vi "DI Block Config Pane.vi"(6 "_SubPanelMessages":refnum<notifier>, 9 "_myEmbeddedToFrameEvent":T7, 10 "_myEmbedded.Exit":refnum<user-event>, 11 "-Property Bundle":cluster{"Name":string, "Value":variant}[](array[cluster])) -> (1 "_Connection Informations":T3, 2 "_Scripter Input":T9)   [LabVIEW 2021]
doc: "Reads values from one or more digital input channels. Use this Express VI to read one or multiple samples for each channel at one time."
uses:
  <vilib>/myRIO/Common/Express VI Framework/xctls/myRIO Channel List/myRIO Channel List.xctl
  <vilib>/myRIO/Common/Express VI Framework/typedefs/Config Pane to Framework Ref.ctl
  <vilib>/myRIO/Common/Express VI Framework/typedefs/Data Validate Ref.ctl
  <vilib>/myRIO/Common/Express VI Framework/typedefs/Scripter Input.ctl
  <vilib>/myRIO/Common/Express VI Framework/typedefs/WireThrough Terminal Names.ctl
  <vilib>/myRIO/Common/Express VI Framework/typedefs/Instrument Driver Method Descriptor Array.ctl
  <vilib>/myRIO/Common/Express VI Framework/typedefs/Instrument Driver Method Descriptor.ctl
  <vilib>/myRIO/Common/Express VI Framework/typedefs/Sub Panel Messages.ctl
  <vilib>/myRIO/Common/Express VI Framework/typedefs/Connection Informations.ctl
  <vilib>/myRIO/Common/Instrument Driver Framework/Utilities/typedefs/Channel Types.ctl
  <vilib>/myRIO/Common/Express VI Framework/vis/Express VI Framework Strings Global.vi
panel:
  out "_learnMoreLatency":string="Gaps exist between sequential n samples acquisitions Learn more"
  out "_learnMoreFrequency":string="Detailed information about valid sample rates for this Express VI.  Learn more"
  in  "_Validate":bool
  in  "Sample Rate:":dbl=1.0 caption="Sample rate:"
  in  "Sample Rate Unit":enum16{"kHz", "MHz"}(ring)
  in  "Samples to Read:":u32=1000 caption="Samples:" min=1 max=10000
  in  "Name:":string="Digital input (n samples)" caption="Node name:"
  in  "Selected Channel List":T1[](xcontrol)=[{"Channel Name"=0, "Channel Alias"="", "Remove Channel"=FALSE, "Index"=0}]
  in  "_Default Alias String":string
  in  "_VI Default Name (Edit and make value default)":string="Digital input (n samples)"
  in  "_WireThrough Info (Edit and make value default)":T4={"WireThrough Top In"="DI (N Samples) Ref In", "WireThrough Bottom In"="error in (no error)", "WireThrough Top Out"="DI (N Samples) Ref Out", "WireThrough Bottom Out"="error out"}
  in  "_Template Array (Edit and make value default)":T5=[{"Function Name"="Smart Open", "VI Path"=path "<vilib>/myRIO/Instrument Drivers/Onboard IO/DI Block/vis", "Script"=TRUE, "Inputs"=[{"name"="Channel Names", "value"=variant, "Config Pane Only"=TRUE, "Build Array"=FALSE, "Bundle Cluster"=FALSE, "Show Term"=FALSE, "alias"=[], "Required Input"=FALSE}], "Outputs"=[], "VI Class"=enum."Open", "Controls Refs[]"=[], "Inline"=FALSE}, {"Function Name"="Open", "VI Path"=path "<vilib>/myRIO/Instrument Drivers/Onboard IO/DI Block/vis", "Script"=FALSE, "Inputs"=[{"name"="Channel Names", "value"=variant, "Config Pane Only"=TRUE, "Build Array"=FALSE, "Bundle Cluster"=FALSE, "Show Term"=FALSE, "alias"=[], "Required Input"=FALSE}], "Outputs"=[], "VI Class"=enum."Open", "Controls Refs[]"=[], "Inline"=FALSE}, {"Function Name"="Read", "VI Path"=path "<vilib>/myRIO/Instrument Drivers/Onboard IO/DI Block/vis", "Script"=TRUE, "Inputs"=[{"name"="Number of Samples", "value"=variant, "Config Pane Only"=TRUE, "Build Array"=FALSE, "Bundle Cluster"=FALSE, "Show Term"=FALSE, "alias"=[], "Required Input"=FALSE}, {"name"="Sample Rate [Hz]", "value"=variant, "Config Pane Only"=TRUE, "Build Array"=FALSE, "Bundle Cluster"=FALSE, "Show Term"=FALSE, "alias"=[], "Required Input"=FALSE}], "Outputs"=[{"name"="Values", "value"=variant, "Show Term"=TRUE, "Index Array"=TRUE, "Unbundle Cluster"=FALSE, "alias"=[]}], "VI Class"=enum."Data", "Controls Refs[]"=[], "Inline"=FALSE}, {"Function Name"="Close", "VI Path"=path "<vilib>/myRIO/Instrument Drivers/Onboard IO/DI Block/vis", "Script"=FALSE, "Inputs"=[], "Outputs"=[], "VI Class"=enum."Close", "Controls Refs[]"=[], "Inline"=FALSE}]
  in  "_Test Close":bool
  # "User Visible Area"
  # "NOTE: Tab Order has been set\nfor this Front Panel.\n1. Name: (string control)\n2. Add Channel (button)\n3. Selected Channel List (array)\n\nAll other controls are excluded \nfrom Tabbing order\n\nTo exlude a control from context\nhelp prefix its label text with a '-'"
  # "Gap:"
  # "Acquired signal"
  # "Missed signal"
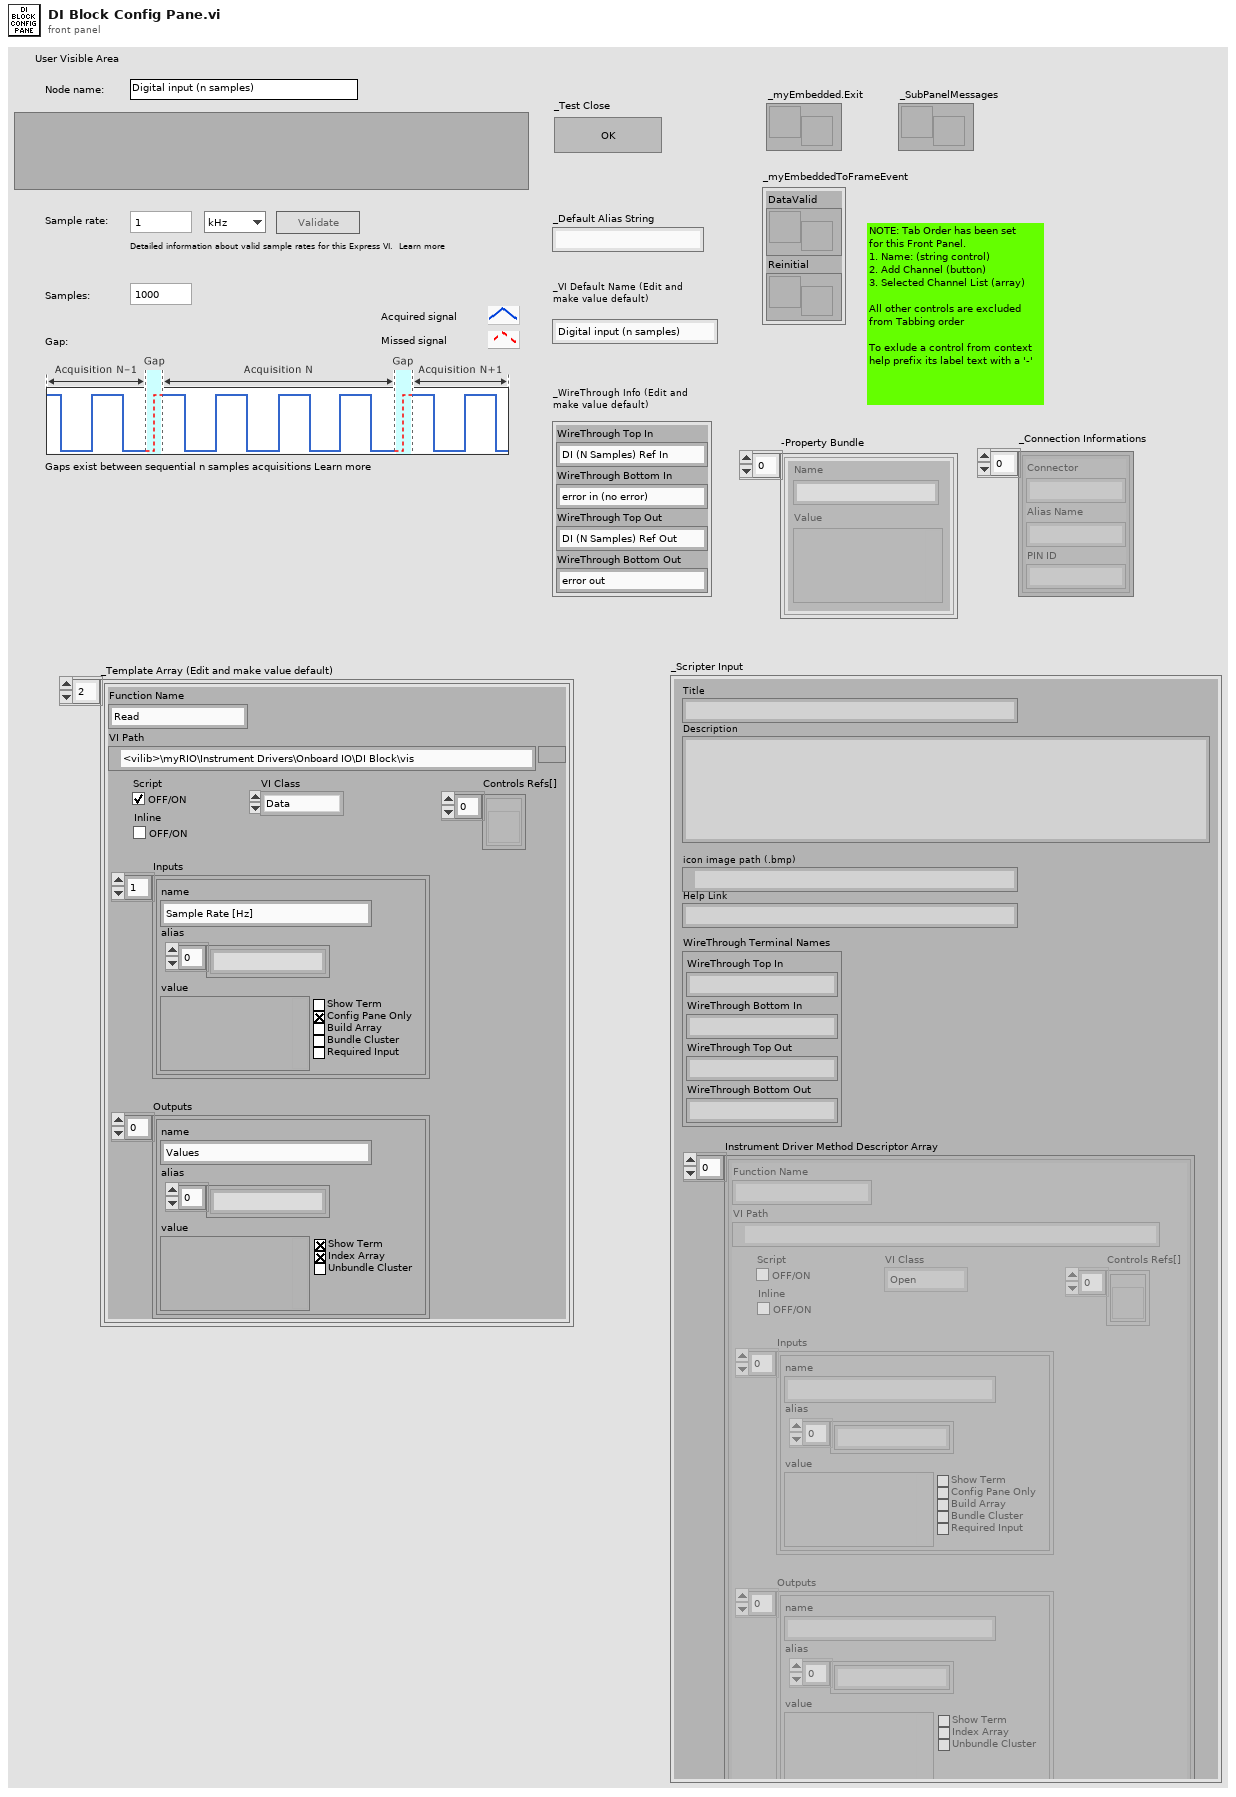
[diagram p1: front panel]
types:
  T1 = typedef "myRIO Channel List.xctl/Channel Data.ctl" = cluster{"Channel Name":u16, "Channel Alias":string, "Remove Channel":T2, "Index":i32}
  T2 = typedef "myRIO Channel List.xctl/Remove Channel.ctl" = bool
  T3 = typedef "Connection Informations.ctl" = cluster{"Connector":string, "Alias Name":string, "PIN ID":string}[]
  T4 = typedef "WireThrough Terminal Names.ctl" = cluster{"WireThrough Top In":string, "WireThrough Bottom In":string, "WireThrough Top Out":string, "WireThrough Bottom Out":string}
  T5 = typedef "Instrument Driver Method Descriptor Array.ctl" = T6[]
  T6 = typedef "Instrument Driver Method Descriptor.ctl" = cluster{"Function Name":string, "VI Path":path, "Script":bool, "Inputs":cluster{"name":string, "value":variant, "Config Pane Only":bool, "Build Array":bool, "Bundle Cluster":bool, "Show Term":bool, "alias":string[], "Required Input":bool}[], "Outputs":cluster{"name":string, "value":variant, "Show Term":bool, "Index Array":bool, "Unbundle Cluster":bool, "alias":string[]}[], "VI Class":enum16{"Open", "Configure", "Data", "Manage", "Close"}, "Controls Refs[]":refnum<vi>[], "Inline":bool}
  T7 = typedef "Config Pane to Framework Ref.ctl" = cluster{"DataValid":T8, "Reinitial":refnum<user-event>}
  T8 = typedef "Data Validate Ref.ctl" = refnum<user-event>
  T9 = typedef "Scripter Input.ctl" = cluster{"Title":string, "Description":string, "icon image path (.bmp)":path, "Help Link":string, "WireThrough Terminal Names":T4, "Instrument Driver Method Descriptor Array":T5}
  T10 = typedef "Channel Types.ctl" = enum32{"Unknown", "AI", "AO", "DIO - DI", "DIO", "DIO - DO", "I2C", "PWM", "Encoder", "SPI", "UART", "Accelerometer", "DIO - LED", "DIO - Button", "AI (N Samples)", "AudioIn (N Samples)", "AO (N Samples)", "AudioOut (N Samples)", "DI (N Samples)", "DO (N Samples)", "AI IRQ", "DI IRQ", "Timer IRQ", "RSL", "Relay", "CAN", "AI (Continuous)", "AO (Continuous)"}
  T11 = typedef "Channel Info.ctl" = cluster{"Channel Name":string, "Alias":string, "Used?":bool, "Not Support?":bool, "Property Bundle":cluster{"Name":string, "Value":variant}[]}
  T12 = typedef "Sub Panel Messages.ctl" = enum16{"Initialized"}
  T13 = enum8{"Enabled", "Disabled", "Disabled and Grayed Out"}
  T14 = cluster{"Connector":string, "Alias Name":string, "PIN ID":string}[]
  T15 = cluster{"name":string, "value":variant, "Config Pane Only":bool, "Build Array":bool, "Bundle Cluster":bool, "Show Term":bool, "alias":string[], "Required Input":bool}[]
  T16 = cluster{"name":string, "value":variant, "Config Pane Only":bool, "Build Array":bool, "Bundle Cluster":bool, "Show Term":bool, "alias":string[], "Required Input":bool}
  T17 = cluster{"name":string, "value":variant, "Show Term":bool, "Index Array":bool, "Unbundle Cluster":bool, "alias":string[]}[]
  T18 = cluster{"name":string, "value":variant, "Show Term":bool, "Index Array":bool, "Unbundle Cluster":bool, "alias":string[]}
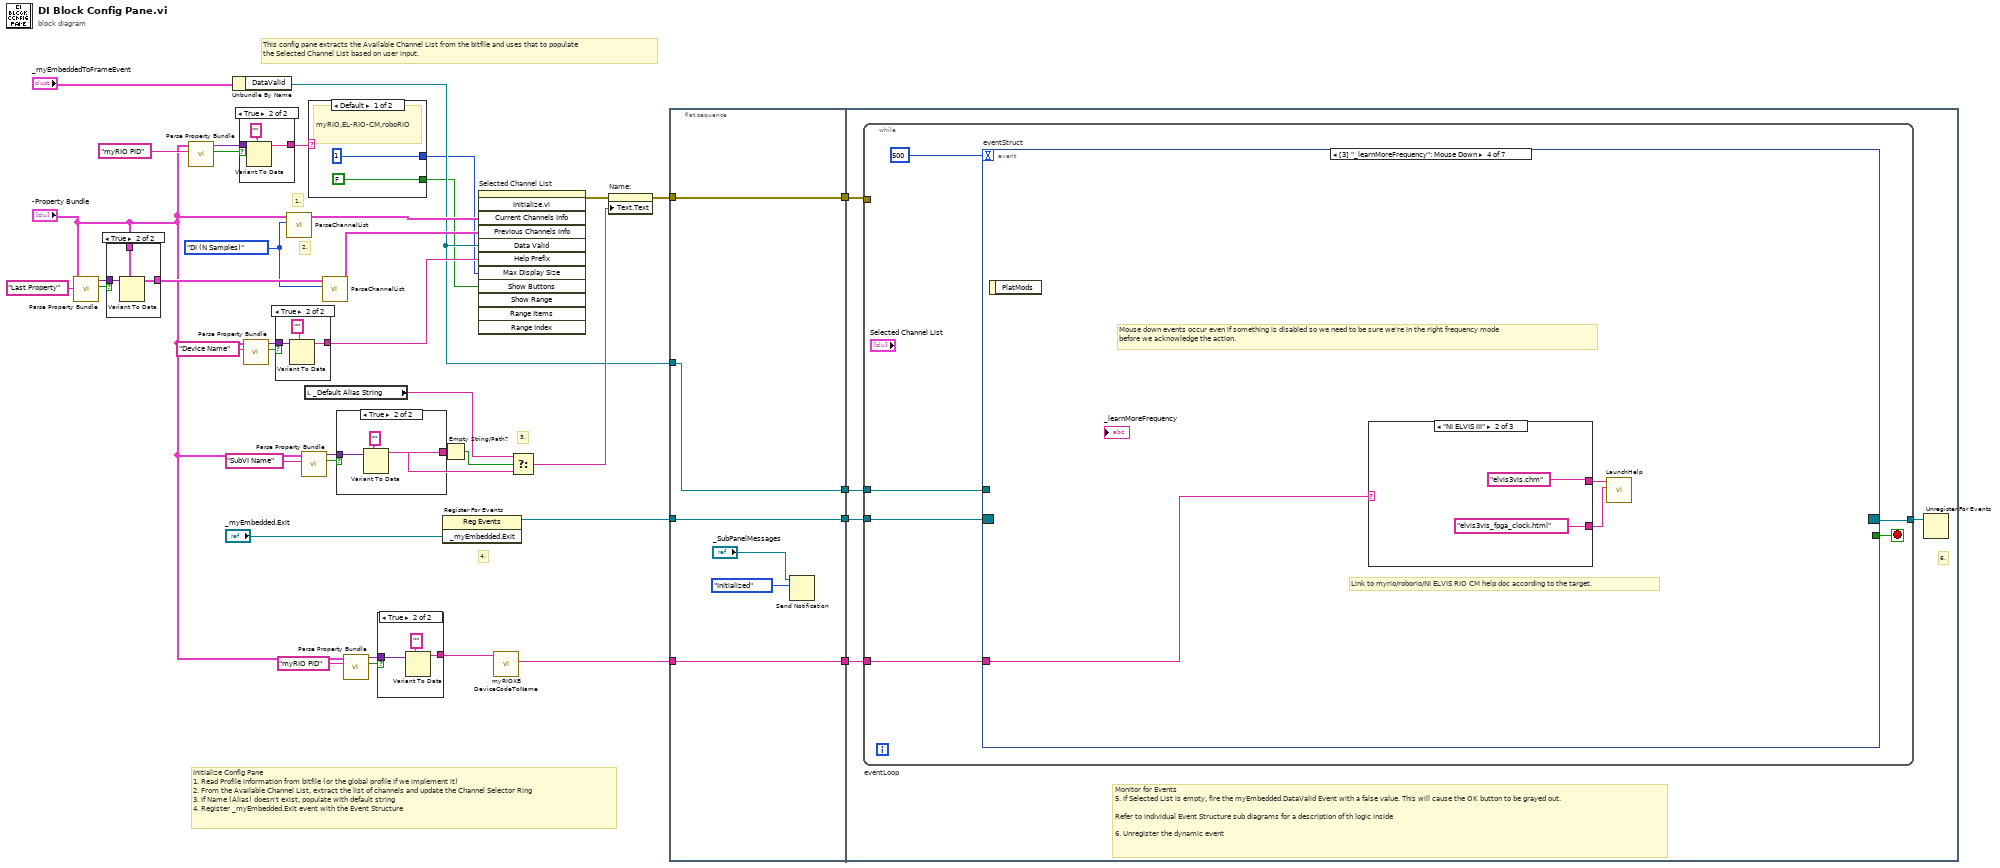
[diagram p0: block diagram]
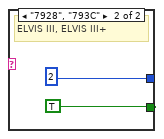
[diagram p2: hidden frame]
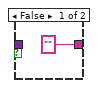
[diagram p3: hidden frame]
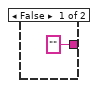
[diagram p4: hidden frame]
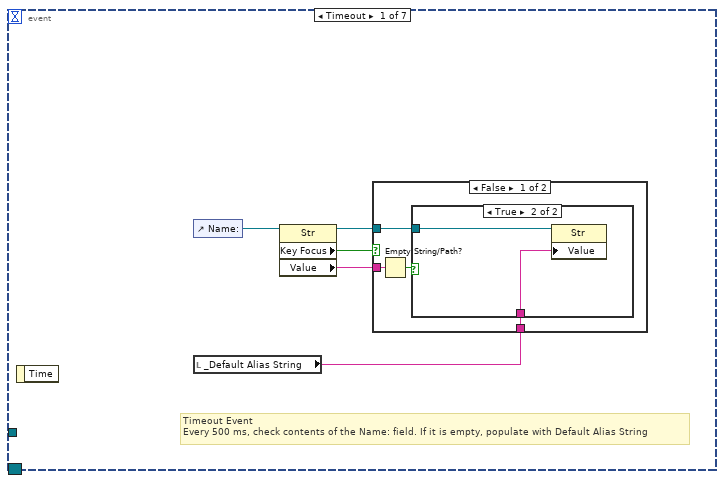
[diagram p5: hidden frame]
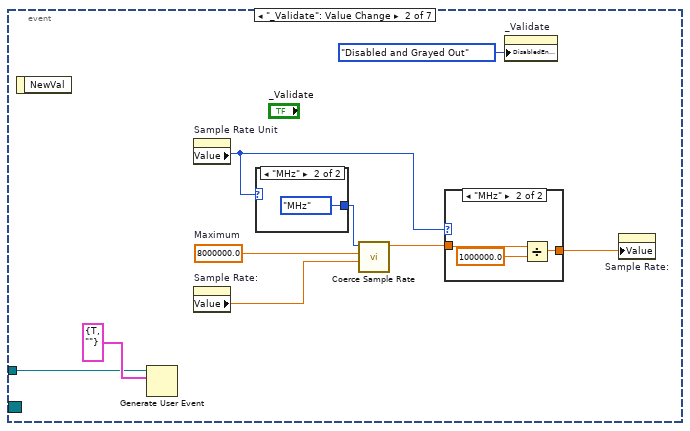
[diagram p8: hidden frame]
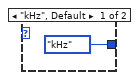
[diagram p9: hidden frame]
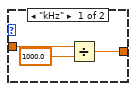
[diagram p10: hidden frame]
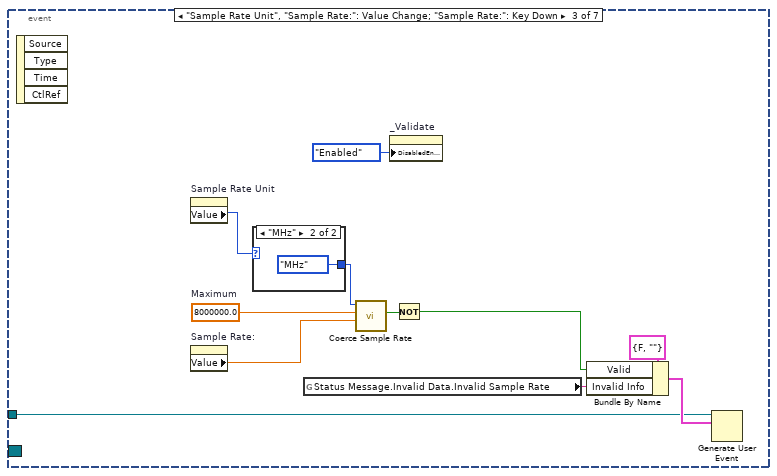
[diagram p11: hidden frame]
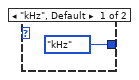
[diagram p12: hidden frame]
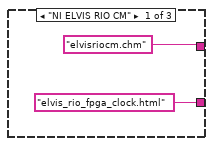
[diagram p13: hidden frame]
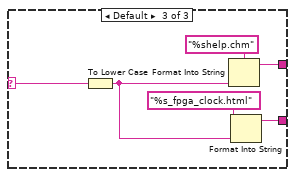
[diagram p14: hidden frame]
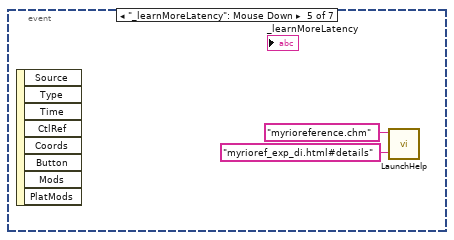
[diagram p15: hidden frame]
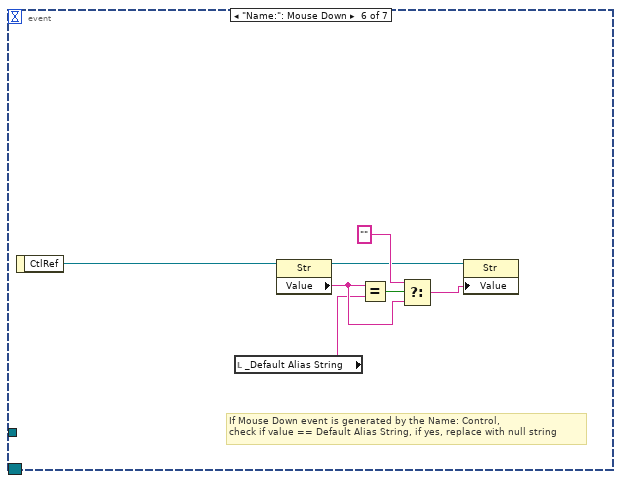
[diagram p16: hidden frame]
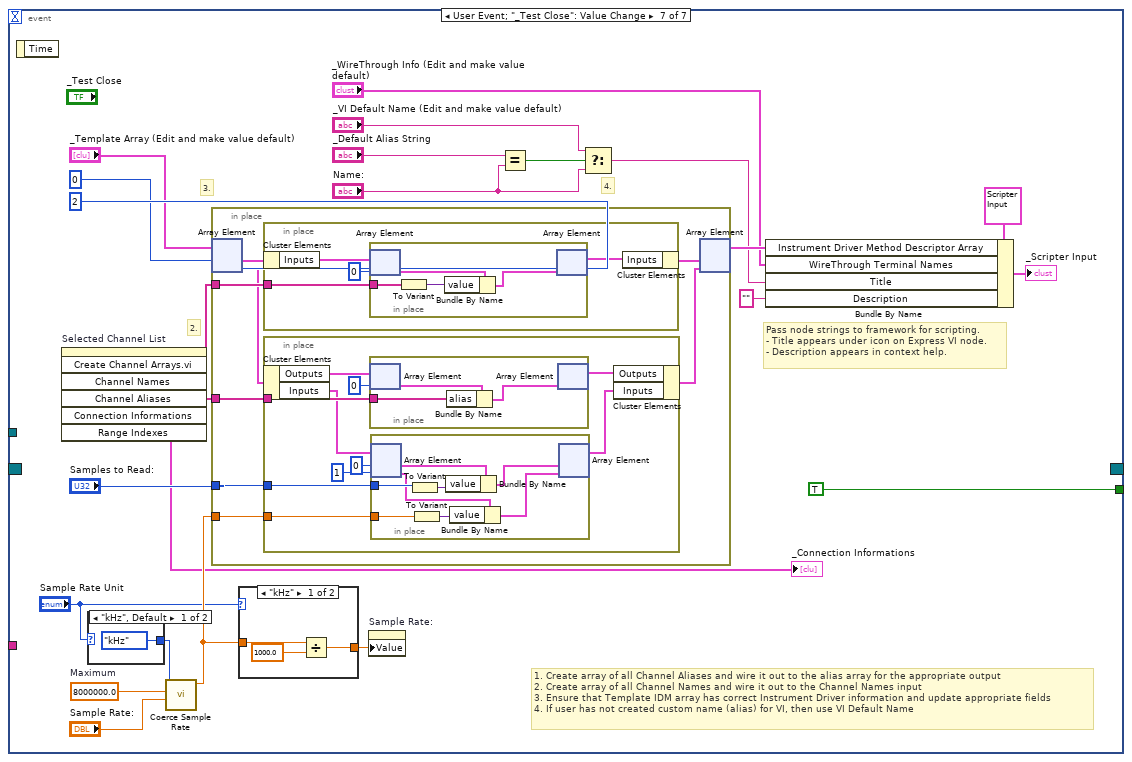
[diagram p17: hidden frame]
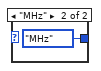
[diagram p18: hidden frame]
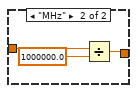
[diagram p19: hidden frame]
diagram:
  w24 = Channel_Types."DI (N Samples)" ("Channel to Read")
  # "This config pane extracts the Available Channel List from the bitfile and uses that to populate\nthe Selected Channel List based on user input."
  # "2."
  # "1."
  # "4."
  # "3."
  # "Initialize Config Pane\n1. Read Profile information from bitfile (or the global profile if we implement it)\n2. From the Available Channel List, extract the list of channels and update the Channel Selector Ring\n3. If Name (Alias) doesn't exist, populate with default string\n4. Register _myEmbedded.Exit event with the Event Structure"
  n1 = call <vilib>:"Parse Property Bundle.vi"("Name"="Last Property", "Property Bundle"="-Property Bundle") -> ("Found?"=w26:bool, "Value"=w27:variant)  [unwired: 8 in]
  n2 = case shown="True" w26 {
    tunnel: w27 -> [_ w43]
    tunnel: [_ w42] -> w25
    tunnel: "-Property Bundle" -> [_ w41]
    frame False {
    }
    frame True {
      n3 = Variant To Data(type=w41, Variant=w43) -> (data=w42:cluster{"Name":string, "Value":variant}[])  [unwired: 1 in, 1 out]
    }
  }
  n4 = call <vilib>:"Parse Property Bundle.vi"("Name"="myRIO PID", "Property Bundle"="-Property Bundle") -> ("Found?"=w5:bool, "Value"=w6:variant)  [unwired: 8 in]
  n5 = Unbundle By Name("_myEmbeddedToFrameEvent") -> ("DataValid"=w15:T8)
  n6 = case shown="True" w5 {
    tunnel: w6 -> [_ w47]
    tunnel: ["" ("Name") w46] -> w4
    frame False {
    }
    frame True {
      n7 = Variant To Data(type="" ("Name"), Variant=w47) -> (data=w46:string)  [unwired: 1 in, 1 out]
    }
  }
  n8 = call <vilib>:"Parse Property Bundle.vi"("Name"="Device Name", "Property Bundle"="-Property Bundle") -> ("Found?"=w21:bool, "Value"=w20:variant)  [unwired: 8 in]
  n9 = case shown="True" w21 {
    tunnel: w20 -> [_ w50]
    tunnel: [_ w49] -> w19
    frame False {
    }
    frame True {
      n10 = Variant To Data(type="", Variant=w50) -> (data=w49:string)  [unwired: 1 in, 1 out]
    }
  }
  n11 = call <vilib>:"ParseChannelList.vi"("Channel to Read"=w24, "_Property Bundle"="-Property Bundle") -> ("Channel List Out"=w29:T11[])  [unwired: 7 in, 2 out]
  n12 = call <vilib>:"Parse Property Bundle.vi"("Name"="SubVI Name", "Property Bundle"="-Property Bundle") -> ("Found?"=w34:bool, "Value"=w35:variant)  [unwired: 8 in]
  n13 = local read "_Default Alias String"() -> (w30:string)
  n14 = case shown="Default" w4 {
    tunnel: [FALSE TRUE] -> w2
    tunnel: [1 ("Max Display Size") 2 ("Max Display Size")] -> w1
    frame Default {
      # "myRIO,EL-RIO-CM,roboRIO"
    }
    frame "7928", "793C" {
      # "ELVIS III, ELVIS III+"
    }
  }
  n15 = call <vilib>:"ParseChannelList.vi"("Channel to Read"=w24, "_Property Bundle"=w25) -> ("Channel List Out"=w23:T11[])  [unwired: 7 in, 2 out]
  n16 = case shown="True" w34 {
    tunnel: w35 -> [_ w58]
    tunnel: ["" ("Name") w56] -> w33
    frame False {
    }
    frame True {
      n17 = Variant To Data(type="" ("Name"), Variant=w58) -> (data=w56:string)  [unwired: 1 in, 1 out]
    }
  }
  n18 = call <vilib>:"Parse Property Bundle.vi"("Name"="myRIO PID", "Property Bundle"="-Property Bundle") -> ("Found?"=w11:bool, "Value"=w12:variant)  [unwired: 8 in]
  n19 = case shown="True" w11 {
    tunnel: w12 -> [_ w62]
    tunnel: ["" ("Name") w60] -> w8
    frame False {
    }
    frame True {
      n20 = Variant To Data(type="" ("Name"), Variant=w62) -> (data=w60:string)  [unwired: 1 in, 1 out]
    }
  }
  n21 = register-events("_myEmbedded.Exit") -> (reference out=w32:refnum<event-registration>)  [unwired: 2 in, 1 out]
  n22 = Empty String/Path?(string/path=w33) -> (empty?=w39:bool)
  n23 = invoke on="Selected Channel List" class="myRIO Channel List (strict)" method="Initialize.vi"("Current Channels Info"=w29, "Previous Channels Info"=w23, "Data Valid"=w15, "Help Prefix"=w19, "Max Display Size"=w1, "Show Buttons"=w2) -> (error out=w31:errorcluster)  [unwired: 6 in, 11 out]
  n24 = call <vilib>:"myRIOXB DeviceCodeToName.vi"("Device Code"=w8) -> ("Name"=w9:string)  [unwired: 10 in]
  n25 = Select(t=w30, s=w39, f=w33) -> (s? t:f=w38:string)
  n26 = property on="Name:" class="Str"(error in=w31, "Text.Text"=w38) -> (error out=w37:errorcluster)  [unwired: 1 in, 1 out]
  n27 = flat-sequence {
    tunnel: w32 -> [w67]
    tunnel: w37 -> [w68]
    tunnel: [w68] -> w17
    tunnel: [w67] -> w16
    tunnel: w15 -> [w64]
    tunnel: [w64] -> w14
    tunnel: w9 -> [w63]
    tunnel: [w63] -> w10
    tunnel: w17 -> [w72]
    tunnel: w16 -> [w71]
    tunnel: w14 -> [w70]
    tunnel: w10 -> [w69]
    frame #0 {
      n28 = Send Notification(notification=Sub_Panel_Messages."Initialized", notifier="_SubPanelMessages") -> ()  [unwired: 1 in, 2 out]
    }
    frame #1 {
      # "6."
      # "Monitor for Events\n5. If Selected List is empty, fire the myEmbedded.DataValid Event with a false value. This will cause the OK button to be grayed out.\n\nRefer to individual Event Structure sub diagrams for a description of th logic inside\n\n6. Unregister the dynamic event"
      n29 = while "eventLoop" {
        tunnel: w71 -> [w78]
        tunnel: [w77] -> w73
        tunnel: w72 -> [_]
        tunnel: w70 -> [w75]
        tunnel: w69 -> [w74]
        stop <- w79 stop-if-true
        n30 = event "eventStruct" shown="[3] \"_learnMoreFrequency\": Mouse Down" {
          selector: w78 -> [_ _ _ _ _ _ _]
          dyn-events: [_ _ _ _ _ _ _] -> w77
          timeout: 500 -> [_ _ _ _ _ _ _]
          tunnel: [_ _ _ _ _ _ TRUE ("_Test Close")] -> w79
          tunnel: w75 -> [_ w91 w110 _ _ _ _]
          tunnel: w74 -> [_ _ _ w121 _ _ _]
          event Timeout {
            # "Timeout Event\nEvery 500 ms, check contents of the Name: field. If it is empty, populate with Default Alias String"
            n31 = event-data() -> ()  [unwired: 1 in, 1 out]
            n32 = control-ref of="Name:"() -> (w82:refnum<vi>)
            n33 = local read "_Default Alias String"() -> (w80:string)
            n34 = property on="Property Node" class="Str"(reference=w82) -> (reference out=w81:refnum<vi>, "Key Focus"=w83:bool, "Value"=w84:string)  [unwired: 1 in, 1 out]
            n35 = case shown="False" w83 {
              tunnel: w84 -> [w88 _]
              tunnel: w81 -> [w86 _]
              tunnel: w80 -> [w85 _]
              frame False {
                n36 = Empty String/Path?(string/path=w88) -> (empty?=w87:bool)
                n37 = case shown="True" w87 {
                  tunnel: w86 -> [_ w90]
                  tunnel: w85 -> [_ w89]
                  frame False {
                  }
                  frame True {
                    n38 = property on="Property Node" class="Str"(reference=w90, "Value"=w89) -> ()  [unwired: 1 in, 2 out]
                  }
                }
              }
              frame True {
              }
            }
          }
          event "_Validate": Value Change {
            w97 = 8000000.0  # Maximum
            n39 = event-data() -> ()  [unwired: 1 in, 1 out]
            n40 = Generate User Event(user event=w91, event data cluster=cluster{"Valid":bool, "Invalid Info":string} {"Valid"=TRUE, "Invalid Info"=""} ("event data")) -> ()  [unwired: 2 in, 2 out]
            n41 = property on="Sample Rate Unit" class="Enum (strict)"() -> ("Value"=w94:enum16{"kHz", "MHz"})  [unwired: 2 in, 2 out]
            n42 = property on="Sample Rate:" class="DigNum (strict)"() -> ("Value"=w96:dbl)  [unwired: 2 in, 2 out]
            n43 = case shown="\"MHz\"" w94 {
              tunnel: [enum16{"Hz", "kHz", "MHz"}."kHz" ("Sample Rate Unit") enum16{"Hz", "kHz", "MHz"}."MHz" ("Sample Rate Unit")] -> w93
              frame "kHz", Default {
              }
              frame "MHz" {
              }
            }
            n44 = call <vilib>:"Coerce Sample Rate.vi"("Sample Rate:"=w96, "Maximum"=w97, "Sample Rate Unit"=w93) -> ("Actual Sample Rate (s)"=w98:dbl)  [unwired: 7 in, 1 out]
            n45 = case shown="\"MHz\"" w94 {
              tunnel: w98 -> [w104 w106]
              tunnel: [w102 w105] -> w95
              frame "kHz" {
                n46 = Divide(x=w104, y=1000.0) -> (x/y=w102:dbl)
              }
              frame "MHz" {
                n47 = Divide(x=w106, y=1000000.0) -> (x/y=w105:dbl)
              }
            }
            n48 = property on="_Validate" class="Bool"("DisabledEnum"=T13."Disabled and Grayed Out" ("Disabled")) -> ()  [unwired: 2 in, 2 out]
            n49 = property on="Sample Rate:" class="DigNum (strict)"("Value"=w95) -> ()  [unwired: 2 in, 2 out]
          }
          event "Sample Rate Unit", "Sample Rate:": Value Change; "Sample Rate:": Key Down {
            w117 = 8000000.0  # Maximum
            n50 = event-data() -> ()  [unwired: 1 in, 4 out]
            n51 = property on="Sample Rate Unit" class="Enum (strict)"() -> ("Value"=w115:enum16{"kHz", "MHz"})  [unwired: 2 in, 2 out]
            n52 = property on="Sample Rate:" class="DigNum (strict)"() -> ("Value"=w116:dbl)  [unwired: 2 in, 2 out]
            n53 = case shown="\"MHz\"" w115 {
              tunnel: [enum16{"Hz", "kHz", "MHz"}."kHz" ("Sample Rate Unit") enum16{"Hz", "kHz", "MHz"}."MHz" ("Sample Rate Unit")] -> w114
              frame "kHz", Default {
              }
              frame "MHz" {
              }
            }
            n54 = global read "Express VI Framework Strings Global.vi" "Status Message.Invalid Data.Invalid Sample Rate"() -> (w111:string)
            n55 = call <vilib>:"Coerce Sample Rate.vi"("Sample Rate:"=w116, "Maximum"=w117, "Sample Rate Unit"=w114) -> ("Coercion needed?"=w109:bool)  [unwired: 7 in, 1 out]
            n56 = property on="_Validate" class="Bool"("DisabledEnum"=T13."Enabled" ("Disabled")) -> ()  [unwired: 2 in, 2 out]
            n57 = Not(x=w109) -> (.not. x?=w108:bool)
            n58 = Bundle By Name(cluster=cluster{"Valid":bool, "Invalid Info":string} {"Valid"=FALSE, "Invalid Info"=""} ("event data"), "Valid"=w108, "Invalid Info"=w111) -> (w112:cluster{"Valid":bool, "Invalid Info":string})
            n59 = Generate User Event(user event=w110, event data cluster=w112) -> ()  [unwired: 2 in, 2 out]
          }
          event "_learnMoreFrequency": Mouse Down {
            # "Link to myrio/roborio/NI ELVIS RIO CM help doc according to the target."
            # "Mouse down events occur even if something is disabled so we need to be sure we're in the right frequency mode\nbefore we acknowledge the action."
            n60 = event-data() -> ()  [unwired: 1 in, 1 out]
            n61 = case shown="\"NI ELVIS III\"" w121 {
              selector: w121 -> [_ _ w128]
              tunnel: ["elvisriocm.chm" ("Help File") "elvis3vis.chm" ("Help File") w130] -> w123
              tunnel: ["elvis_rio_fpga_clock.html" ("Help Topic") "elvis3vis_fpga_clock.html" ("Help Topic") w129] -> w122
              frame "NI ELVIS RIO CM" {
              }
              frame "NI ELVIS III" {
              }
              frame Default {
                n62 = To Lower Case(string=w128) -> (all lower case string=w132:string)
                n63 = Format Into String(format string="%shelp.chm" ("Help File"), w132) -> (resulting string=w130:string)  [unwired: 2 in, 1 out]
                n64 = Format Into String(format string="%s_fpga_clock.html" ("Help Topic"), w132) -> (resulting string=w129:string)  [unwired: 2 in, 1 out]
              }
            }
            n65 = call <vilib>:"LaunchHelp.vi"("Help Topic"=w122, "Help File"=w123) -> ()  [unwired: 10 in]
          }
          event "_learnMoreLatency": Mouse Down {
            n66 = event-data() -> ()  [unwired: 1 in, 8 out]
            n67 = call <vilib>:"LaunchHelp.vi"("Help Topic"="myrioref_exp_di.html#details", "Help File"="myrioreference.chm") -> ()  [unwired: 10 in]
          }
          event "Name:": Mouse Down {
            # "If Mouse Down event is generated by the Name: Control,\ncheck if value == Default Alias String, if yes, replace with null string"
            n68 = event-data() -> ("CtlRef"=w142:refnum<vi>)  [unwired: 1 in]
            n69 = local read "_Default Alias String"() -> (w136:string)
            n70 = property class="Str"(reference=w142) -> (reference out=w138:refnum<vi>, "Value"=w137:string)  [unwired: 1 in, 1 out]
            n71 = Equal?(x=w137, y=w136) -> (x = y?=w141:bool)
            n72 = Select(t="", s=w141, f=w137) -> (s? t:f=w139:string)
            n73 = property class="Str"(reference=w138, "Value"=w139) -> ()  [unwired: 1 in, 2 out]
          }
          event User Event; "_Test Close": Value Change {
            w149 = 8000000.0  # Maximum
            # "1."
            # "2."
            # "1. Create array of all Channel Aliases and wire it out to the alias array for the appropriate output\n2. Create array of all Channel Names and wire it out to the Channel Names input\n3. Ensure that Template IDM array has correct Instrument Driver information and update appropriate fields\n4. If user has not created custom name (alias) for VI, then use VI Default Name"
            # "4."
            # "3."
            # "Pass node strings to framework for scripting.\n- Title appears under icon on Express VI node.\n- Description appears in context help."
            n74 = event-data() -> ()  [unwired: 1 in, 1 out]
            n75 = invoke on="Selected Channel List" class="myRIO Channel List (strict)" method="Create Channel Arrays.vi"() -> ("Channel Names"=w146:string[], "Channel Aliases"=w147:string[], "Connection Informations"=→"_Connection Informations":T14)  [unwired: 7 in, 4 out]
            n76 = case shown="\"kHz\", Default" "Sample Rate Unit" {
              tunnel: [enum16{"Hz", "kHz", "MHz"}."kHz" ("Sample Rate Unit") enum16{"Hz", "kHz", "MHz"}."MHz" ("Sample Rate Unit")] -> w143
              frame "kHz", Default {
              }
              frame "MHz" {
              }
            }
            n77 = call <vilib>:"Coerce Sample Rate.vi"("Sample Rate:"="Sample Rate:", "Maximum"=w149, "Sample Rate Unit"=w143) -> ("Actual Sample Rate (s)"=w148:dbl)  [unwired: 7 in, 1 out]
            n78 = in-place {
              in-place-border: w146 -> [w179]
              in-place-border: w147 -> [w178]
              in-place-border: "Samples to Read:" -> [w176]
              in-place-border: w148 -> [w175]
              n79 = in-place-array #1("_Template Array (Edit and make value default)", 0, 2) -> (w182:T6, w177:T6)
              n80 = in-place {
                in-place-border: w179 -> [w206]
                n81 = in-place-cluster #2(w182) -> ("Inputs"=w207:T15)
                n82 = in-place {
                  in-place-border: w206 -> [w208]
                  n83 = in-place-array #3(w207, 0) -> (w211:T16)
                  n84 = To Variant(anything=w208) -> (Variant=w209:variant)
                  n85 = Bundle By Name(cluster=w211, "value"=w209) -> (w210:T16)
                  n86 = in-place-array #3(w210) -> (w205:T15)  [unwired: 1 out]
                }
                n87 = in-place-cluster #2("Inputs"=w205) -> (w181:T6)
              }
              n88 = in-place {
                in-place-border: w178 -> [w191]
                in-place-border: w176 -> [w185]
                in-place-border: w175 -> [w184]
                n89 = in-place-cluster #4(w177) -> ("Outputs"=w192:T17, "Inputs"=w188:T15)
                n90 = in-place {
                  in-place-border: w191 -> [w201]
                  n91 = in-place-array #5(w192, 0) -> (w203:T18)
                  n92 = Bundle By Name(cluster=w203, "alias"=w201) -> (w202:T18)
                  n93 = in-place-array #5(w202) -> (w190:T17)  [unwired: 1 out]
                }
                n94 = in-place {
                  in-place-border: w185 -> [w198]
                  in-place-border: w184 -> [w195]
                  n95 = in-place-array #6(w188, 0, 1) -> (w200:T16, w196:T16)
                  n96 = To Variant(anything=w198) -> (Variant=w197:variant)
                  n97 = To Variant(anything=w195) -> (Variant=w194:variant)
                  n98 = Bundle By Name(cluster=w200, "value"=w197) -> (w199:T16)
                  n99 = Bundle By Name(cluster=w196, "value"=w194) -> (w193:T16)
                  n100 = in-place-array #6(w199, w193) -> (w187:T15)  [unwired: 2 out]
                }
                n101 = in-place-cluster #4("Outputs"=w190, "Inputs"=w187) -> (w180:T6)
              }
              n102 = in-place-array #1(w181, w180) -> (w164:T5)  [unwired: 2 out]
            }
            n103 = case shown="\"kHz\"" "Sample Rate Unit" {
              tunnel: w148 -> [w171 w173]
              tunnel: [w169 w172] -> w151
              frame "kHz" {
                n104 = Divide(x=w171, y=1000.0) -> (x/y=w169:dbl)
              }
              frame "MHz" {
                n105 = Divide(x=w173, y=1000000.0) -> (x/y=w172:dbl)
              }
            }
            n106 = property on="Sample Rate:" class="DigNum (strict)"("Value"=w151) -> ()  [unwired: 2 in, 2 out]
            n107 = Equal?(x="_Default Alias String", y="Name:") -> (x = y?=w156:bool)
            n108 = Select(t="_VI Default Name (Edit and make value default)", s=w156, f="Name:") -> (s? t:f=w154:string)
            n109 = Bundle By Name(cluster=T9 {"Title"="", "Description"="", "icon image path (.bmp)"=path "", "Help Link"="", "WireThrough Terminal Names"={"WireThrough Top In"="", "WireThrough Bottom In"="", "WireThrough Top Out"="", "WireThrough Bottom Out"=""}, "Instrument Driver Method Descriptor Array"=[]} ("Scripter Input"), "Instrument Driver Method Descriptor Array"=w164, "WireThrough Terminal Names"="_WireThrough Info (Edit and make value default)", "Title"=w154, "Description"="" ("Title")) -> (→"_Scripter Input":T9)
          }
        }
      }
      n110 = Unregister For Events(event registration refnum=w73) -> ()  [unwired: 1 in, 1 out]
    }
  }
